vi "Get Column Datatype.vi"(8 "error in (no error)":errorcluster, 9 "Column Name":string, 10 "Table Path":string, 11 "LV-Data.PGSQL in":refnum<class "LV-Data.PGSQL.lvclass">) -> (0 "error out":errorcluster, 2 "Datatype":string, 3 "LV-Data.PGSQL out":refnum<class "LV-Data.PGSQL.lvclass">)   [LabVIEW 2019, in "LV-Data.PGSQL.lvclass"]
uses:
  LV-Data.PGSQL.lvclass
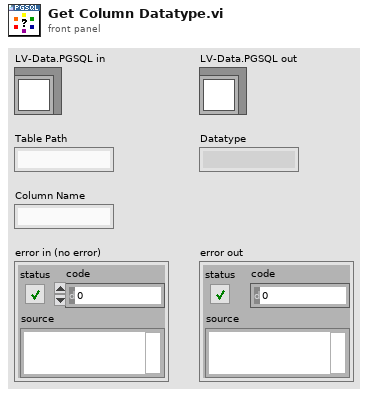
[diagram p1: front panel]
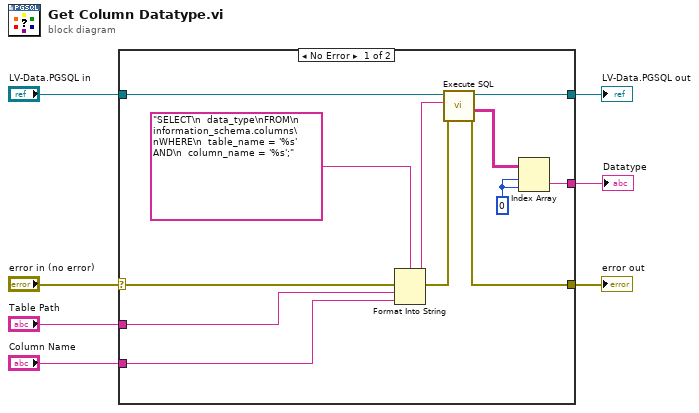
[diagram p0: block diagram]
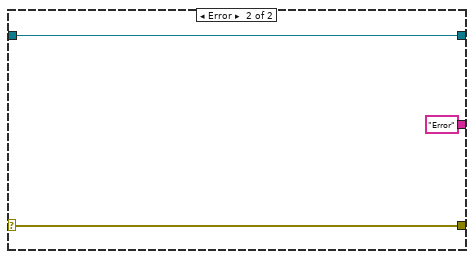
[diagram p2: hidden frame]
diagram:
  n1 = case shown="No Error" "error in (no error)" {
    selector: "error in (no error)" -> [w15 w22]
    tunnel: "Column Name" -> [w16 _]
    tunnel: [w13 w22] -> w7
    tunnel: [w14 w20] -> w5
    tunnel: "Table Path" -> [w17 _]
    tunnel: [w12 "Error" ("Get:Get String")] -> w2
    tunnel: "LV-Data.PGSQL in" -> [w11 w20]
    frame No Error {
      w19 = 0 ("index (row)")
      n2 = Format Into String(format string="SELECT\n  data_type\nFROM\n  information_schema.columns\nWHERE\n  table_name = '%s' AND\n  column_name = '%s';", error in=w15, w17, w16) -> (resulting string=w10:string, error out=w18:errorcluster)  [unwired: 1 in]
      n3 = call "Execute SQL.vi"("error in"=w18, "SQL"=w10, "LV-Data.PGSQL"=w11) -> ("error out"=w13:errorcluster, "Result"=w8:string[][], "LV-Data.PGSQL out"=w14:refnum<class "LV-Data.PGSQL.lvclass">)  [unwired: 5 in, 1 out]
      n4 = Index Array(array=w8, index (row)=w19, index (col)=w19) -> (element=w12:string)
    }
    frame Error {
    }
  }
  "error out" <- w7
  "LV-Data.PGSQL out" <- w5
  "Datatype" <- w2
